vi "test_VI.vi"() -> ()   [LabVIEW 2019]
panel:
  in  "Buttons In":bool[](array[boolean])
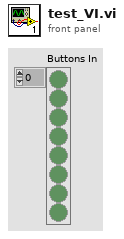
[diagram p1: front panel]
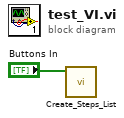
[diagram p0: block diagram]
diagram:
  n1 = call "Create_Steps_List.vi"("Buttons In"="Buttons In") -> ()  [unwired: 10 in, 1 out]
